vi "Agitator Status.vi"() -> ()   [LabVIEW 2021]
uses:
  Controls/Agitator.ctl
panel:
  out "Agitator":T1
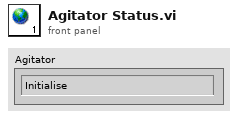
[diagram p1: front panel]
types:
  T1 = typedef "Agitator.ctl" = enum16{"Initialise", "CYL Fwd", "Wait for Delay", "CYL Rear", "Wait For Rest", "Done", "Error"}
diagram:
